vi "Universal DMM User Interface.vi"() -> ()   [LabVIEW 2020]
uses:
  Interface 1/rwr_Read Measurement Reply.ctl
  Workers/Fluke DMM/Fluke DMM.lvclass
  Interface 1/Interface 1.lvclass
  Workers/Keithley DMM/Keithley DMM.lvclass
panel:
  in  "stop 2":bool
  out "Reply Data out 2":T1
  out "Reply Data out":T1
  in  "stop":bool
  # "FLUKE"
  # "KEITHLEY"
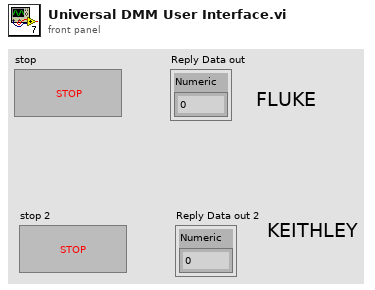
[diagram p1: front panel]
types:
  T1 = typedef "Interface 1.lvclass/rwr_Read Measurement Reply.ctl" = cluster{"Numeric":dbl}
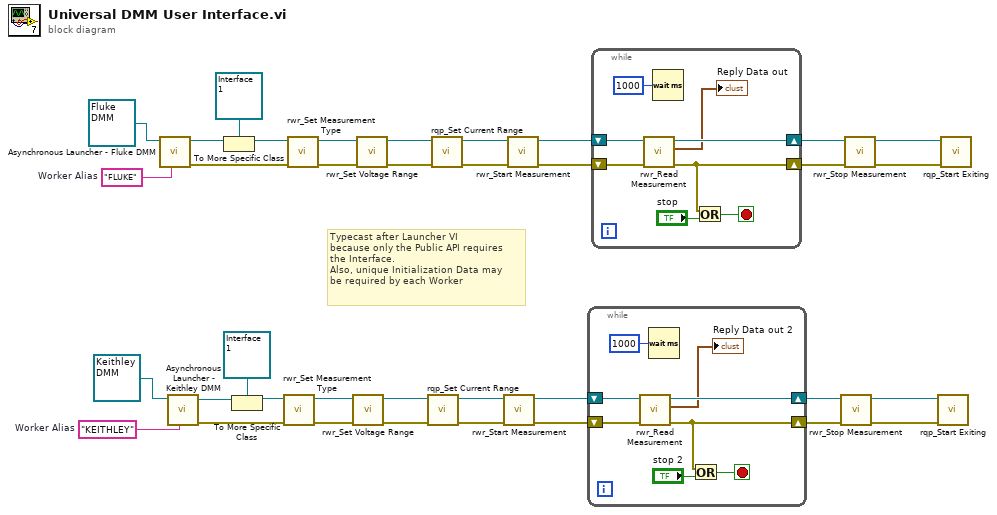
[diagram p0: block diagram]
diagram:
  w8 = "KEITHLEY"  # Worker Alias
  w28 = "FLUKE"  # Worker Alias
  # "Typecast after Launcher VI\nbecause only the Public API requires \nthe Interface.\nAlso, unique Initialization Data may \nbe required by each Worker"
  n1 = call-dynamic "Asynchronous Launcher - Fluke DMM.vi"("Worker Alias"=w28, "Fluke DMM in"=refnum<class "Fluke DMM.lvclass"> refnum ("Fluke DMM")) -> ("error out"=w29:errorcluster, "Fluke DMM out"=w30:refnum<class "Fluke DMM.lvclass">)  [unwired: 8 in]
  n2 = call-dynamic "Asynchronous Launcher - Keithley DMM.vi"("Worker Alias"=w8, "Fluke DMM in"=refnum<class "Keithley DMM.lvclass"> refnum ("Fluke DMM")) -> ("error out"=w15:errorcluster, "Fluke DMM out"=w2:refnum<class "Keithley DMM.lvclass">)  [unwired: 8 in]
  n3 = To More Specific Class(target class=refnum<class "Interface 1.lvclass"> refnum ("Interface 1.lvclass"), reference=w30) -> (specific class reference=w6:refnum<class "Interface 1.lvclass">)  [unwired: 1 in, 1 out]
  n4 = To More Specific Class(target class=refnum<class "Interface 1.lvclass"> refnum ("Interface 1.lvclass"), reference=w2) -> (specific class reference=w3:refnum<class "Interface 1.lvclass">)  [unwired: 1 in, 1 out]
  n5 = call-dynamic "rwr_Set Measurement Type.vi"("error in"=w15, "DMM HAL in"=w3) -> ("error out"=w17:errorcluster, "dup DMM HAL out"=w16:refnum<class "Interface 1.lvclass">)  [unwired: 7 in, 1 out]
  n6 = call-dynamic "rwr_Set Measurement Type.vi"("error in"=w29, "DMM HAL in"=w6) -> ("error out"=w26:errorcluster, "dup DMM HAL out"=w27:refnum<class "Interface 1.lvclass">)  [unwired: 7 in, 1 out]
  n7 = call-dynamic "rwr_Set Voltage Range.vi"("error in"=w17, "DMM HAL in"=w16) -> ("error out"=w18:errorcluster, "dup DMM HAL out"=w20:refnum<class "Interface 1.lvclass">)  [unwired: 7 in, 1 out]
  n8 = call-dynamic "rwr_Set Voltage Range.vi"("error in"=w26, "DMM HAL in"=w27) -> ("error out"=w25:errorcluster, "dup DMM HAL out"=w23:refnum<class "Interface 1.lvclass">)  [unwired: 7 in, 1 out]
  n9 = call-dynamic "rqp_Set Current Range.vi"("error in"=w18, "DMM HAL in"=w20) -> ("error out"=w19:errorcluster, "dup DMM HAL out"=w21:refnum<class "Interface 1.lvclass">)  [unwired: 8 in]
  n10 = call-dynamic "rqp_Set Current Range.vi"("error in"=w25, "DMM HAL in"=w23) -> ("error out"=w24:errorcluster, "dup DMM HAL out"=w22:refnum<class "Interface 1.lvclass">)  [unwired: 8 in]
  n11 = call-dynamic "rwr_Start Measurement.vi"("error in"=w19, "DMM HAL in"=w21) -> ("error out"=w10:errorcluster, "dup DMM HAL out"=w9:refnum<class "Interface 1.lvclass">)  [unwired: 7 in, 1 out]
  n12 = call-dynamic "rwr_Start Measurement.vi"("error in"=w24, "DMM HAL in"=w22) -> ("error out"=w35:errorcluster, "dup DMM HAL out"=w36:refnum<class "Interface 1.lvclass">)  [unwired: 7 in, 1 out]
  n13 = while {
    shift-right: [w42] -> w11
    shift-left: w9 -> [w44]
    shift-right: [w40] -> w12
    shift-left: w10 -> [w43]
    stop <- w39 stop-if-true
    n14 = call-dynamic "rwr_Read Measurement.vi"("error in"=w43, "DMM HAL in"=w44) -> ("error out"=w40:errorcluster, "Reply Data out"=→"Reply Data out 2":T1, "dup DMM HAL out"=w42:refnum<class "Interface 1.lvclass">)  [unwired: 7 in]
    n15 = Wait (ms)(milliseconds to wait=u32 1000) -> ()  [unwired: 1 out]
    n16 = Or(x=w40, y="stop 2") -> (x .or. y?=w39:bool)
  }
  n17 = while {
    shift-right: [w50] -> w34
    shift-left: w36 -> [w52]
    shift-right: [w48] -> w33
    shift-left: w35 -> [w51]
    stop <- w47 stop-if-true
    n18 = call-dynamic "rwr_Read Measurement.vi"("error in"=w51, "DMM HAL in"=w52) -> ("error out"=w48:errorcluster, "Reply Data out"=→"Reply Data out":T1, "dup DMM HAL out"=w50:refnum<class "Interface 1.lvclass">)  [unwired: 7 in]
    n19 = Wait (ms)(milliseconds to wait=u32 1000) -> ()  [unwired: 1 out]
    n20 = Or(x=w48, y="stop") -> (x .or. y?=w47:bool)
  }
  n21 = call-dynamic "rwr_Stop Measurement.vi"("error in"=w12, "DMM HAL in"=w11) -> ("error out"=w14:errorcluster, "dup DMM HAL out"=w13:refnum<class "Interface 1.lvclass">)  [unwired: 7 in, 1 out]
  n22 = call-dynamic "rwr_Stop Measurement.vi"("error in"=w33, "DMM HAL in"=w34) -> ("error out"=w31:errorcluster, "dup DMM HAL out"=w32:refnum<class "Interface 1.lvclass">)  [unwired: 7 in, 1 out]
  n23 = call-dynamic "rqp_Start Exiting.vi"("error in"=w14, "DMM HAL in"=w13) -> ()  [unwired: 8 in, 2 out]
  n24 = call-dynamic "rqp_Start Exiting.vi"("error in"=w31, "DMM HAL in"=w32) -> ()  [unwired: 8 in, 2 out]
